vi "ShapeOK.vi"() -> ()   [LabVIEW 2014]
doc: "This example performs a serial port write and a serial port read. The parameters set for the serial port must match the parameters of the connected instrument or device. The VISA Configure Serial Port VI sets the configuration parameters. The front panel displays the controls used to configure the basic parameters, such as baud rate, data bits, and parity. The VI passes the VISA resource name to other VIs that perform operations on that VISA resource. The VISA Write function sends a command to the serial device and the VISA Read function returns data based on the command. The VISA Close function then closes the reference to the serial device. It is important to close the reference; otherwise, further communication through that port might not be possible."
uses:
  School/MultiSim/LabVIEW 2014/examples/Instrument IO/Serial/support/Serial - Settings.ctl
  HeadControl.ctl
  <vilib>/Instr/_visa.llb/VISA Configure Serial Port (Instr).vi
panel:
  out "HeadPosition":cluster{"X":i16, "Y":i16, "Z":i16}
  in  "MoveHead":T1
  out "Serial Settings:Number of Bytes at Serial Port":u32
  in  "Stop":bool
  in  "Command":string="*IDN?\n"
  in  "Verstuur":bool
  out "Response":string
  out "error out":errorcluster
  in  "Serial Settings":T2={"baud rate"=9600, "data bits"=8, "parity"=enum."None", "stop bits"=10, "flow control"=0} {"flow control" items=["None"=0, "XON/XOFF"=1, "RTS/CTS"=2, "DTR/DSR"=4]; "stop bits" items=["1.0"=10, "1.5"=15, "2.0"=20]; "data bits" min=5 max=8 step=1; "baud rate" items=["75"=75, "110"=110, "134"=134, "150"=150, "300"=300, "600"=600, "1200"=1200, "1800"=1800, "2400"=2400, "4800"=4800, "7200"=7200, "9600"=9600, "14400"=14400, "19200"=19200, "28800"=28800, "38400"=38400, "56000"=56000, "57600"=57600, "115200"=115200, "128000"=128000, "230400"=230400]}
  in  "VISA resource name":refnum<visa-resource-name>="COM1"
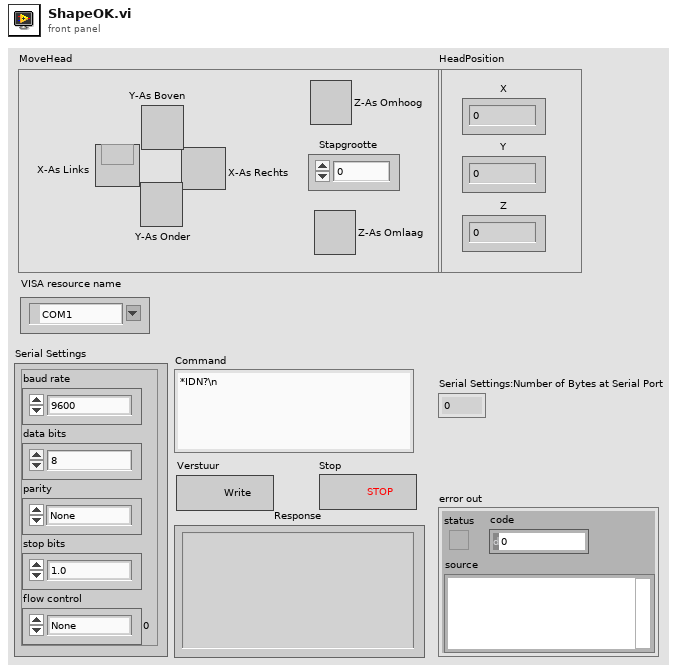
[diagram p1: front panel]
types:
  T1 = typedef "HeadControl.ctl" = cluster{"X-As Links":bool, "X-As Rechts":bool, "Y-As Boven":bool, "Y-As Onder":bool, "Z-As Omhoog":bool, "Z-As Omlaag":bool, "Stapgrootte":i8}
  T2 = typedef "Serial - Settings.ctl" = cluster{"baud rate":u32, "data bits":u16, "parity":enum16{"None", "Odd", "Even", "Mark", "Space"}, "stop bits":u16, "flow control":u16}
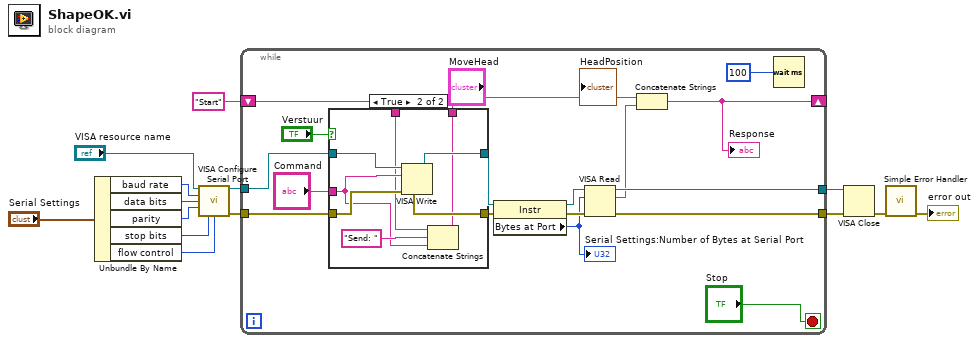
[diagram p0: block diagram]
diagram:
  n1 = Unbundle By Name("Serial Settings") -> ("baud rate"=w12:u32, "data bits"=w11:u16, "parity"=w10:enum16{"None", "Odd", "Even", "Mark", "Space"}, "stop bits"=w9:u16, "flow control"=w8:u16)
  n2 = call-poly "VISA Configure Serial Port"("VISA resource name"="VISA resource name", "baud rate (9600)"=w12, "data bits (8)"=w11, "parity (0:none)"=w10, "stop bits (10: 1 bit)"=w9, "flow control (0:none)"=w8) -> ("VISA resource name out"=w3:refnum<visa-resource-name>, "error out"=w2:errorcluster)  [unwired: 3 in, 5 out]
  n3 = while {
    tunnel: w3 -> [w29]
    tunnel: w2 -> [w28]
    tunnel: [w30] -> w7
    tunnel: [w31] -> w6
    shift-right: [w17] -> _
    shift-left: "Start" -> [w16]
    stop <- "Stop" stop-if-true
    n4 = case shown="True" "Verstuur" {
      tunnel: w29 -> [w34 w42]
      tunnel: w28 -> [w33 w41]
      tunnel: [w34 w39] -> w19
      tunnel: [w33 w40] -> w23
      tunnel: "Command" -> [_ w37]
      tunnel: w16 -> [w32 w36]
      tunnel: [w32 w35] -> w15
      frame False {
      }
      frame True {
        n5 = VISA Write(VISA resource name=w42, write buffer=w37, error in (no error)=w41) -> (VISA resource name out=w39:refnum<visa-resource-name>, error out=w40:errorcluster)  [unwired: 1 out]
        n6 = Concatenate Strings(w36, "Send: ", w37) -> (w35:string)
      }
    }
    n7 = property class="Instr"(reference=w19, error in=w23) -> (reference out=w22:refnum<visa-resource-name>, error out=w21:errorcluster, "Bytes at Port"=w20:u32)
    "Serial Settings:Number of Bytes at Serial Port" <- w20
    n8 = VISA Read(VISA resource name=w22, byte count=w20, error in (no error)=w21) -> (VISA resource name out=w30:refnum<visa-resource-name>, read buffer=w18:string, error out=w31:errorcluster)  [unwired: 1 out]
    n9 = Concatenate Strings(w15, w18) -> (w17:string)
    "Response" <- w17
    n10 = Wait (ms)(milliseconds to wait=u32 100) -> ()  [unwired: 1 out]
  }
  n11 = VISA Close(VISA resource name=w7, error in (no error)=w6) -> (error out=w5:errorcluster)
  n12 = call <vilib>:"Simple Error Handler.vi"("error in (no error)"=w5) -> ("error out"=→"error out":errorcluster)  [unwired: 4 in, 4 out]
